vi "SetParam.vi"(8 "error in (no error)":errorcluster caption="entrée d'erreur (pas d'erreur)", 10 "fetch_covtype":T1={"download_if_missing"=TRUE, "random_state"=-1, "shuffle"=TRUE, "Returns"="Data"} {"random_state" min=-1}, 11 "Covtype.lvclass":refnum<class "Covtype.lvclass">) -> (0 "error out":errorcluster caption="sortie d'erreur", 3 "Covtype.lvclass":refnum<class "Covtype.lvclass">)   [LabVIEW 2020, in "Covtype.lvclass"]
doc: "Set Parameters"
uses:
  Covtype.lvclass
  Covtype.lvclass/Covtype.ctl
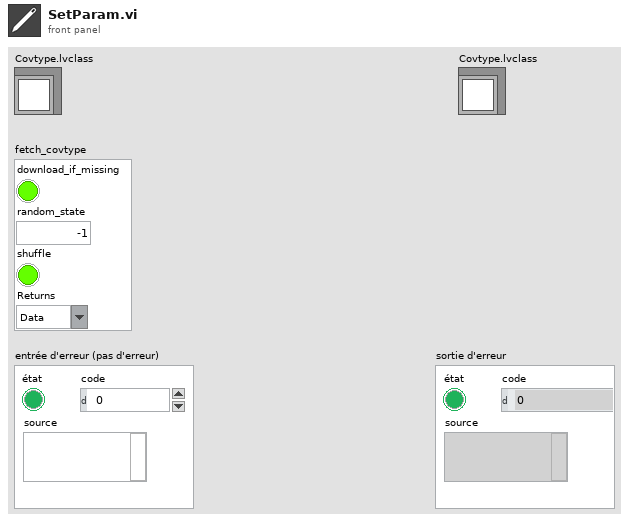
[diagram p1: front panel]
types:
  T1 = cluster{"download_if_missing":bool, "random_state":i32, "shuffle":bool, "Returns":string}
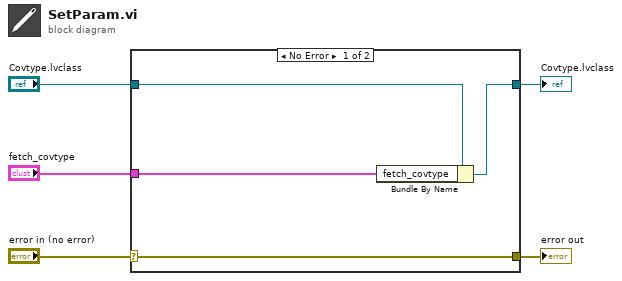
[diagram p0: block diagram]
diagram:
  n1 = case shown="No Error" "error in (no error)" {
    selector: "error in (no error)" -> [w9 w10]
    tunnel: [w9 w10] -> w4
    tunnel: [w7 w11] -> w2
    tunnel: "Covtype.lvclass" -> [w8 w11]
    tunnel: "fetch_covtype" -> [w6 _]
    frame No Error {
      n2 = Bundle By Name(cluster=w8, "fetch_covtype"=w6) -> (w7:refnum<class "Covtype.lvclass">)
    }
    frame Error {
    }
  }
  "error out" <- w4
  "Covtype.lvclass" <- w2
